vi "Read SlavesID.vi"(8 "error in (no error)":errorcluster, 11 "Master in":refnum<class "Master.lvclass">) -> (0 "error out":errorcluster, 2 "SlavesID":i32[](array[numeric]), 3 "Master out":refnum<class "Master.lvclass">)   [LabVIEW 2021, in "Master.lvlib" / "Master.lvclass"]
uses:
  Master.lvclass
  Master.lvclass/Master.ctl
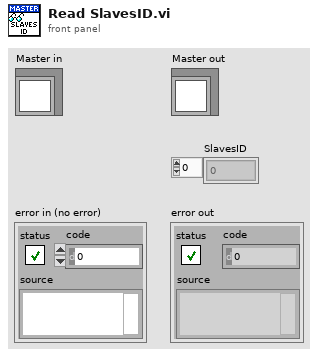
[diagram p1: front panel]
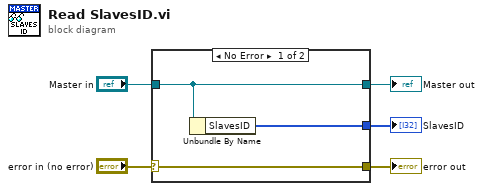
[diagram p0: block diagram]
diagram:
  n1 = case shown="No Error" "error in (no error)" {
    selector: "error in (no error)" -> [w8 w9]
    tunnel: [w8 w9] -> w4
    tunnel: [w7 w10] -> w2
    tunnel: "Master in" -> [w7 w10]
    tunnel: [w6 _] -> w1
    frame No Error {
      n2 = Unbundle By Name(w7) -> ("SlavesID"=w6:i32[])
    }
    frame Error {
    }
  }
  "error out" <- w4
  "Master out" <- w2
  "SlavesID" <- w1
